vi "ADCP main.vi"() -> ()   [LabVIEW 2016, in "ADCP.lvlib"]
uses:
  ADCP.lvlib
  <vilib>/Utility/config.llb/NI_LVConfig.lvlib
panel:
  out "电压串口号":string
  out "电压通信":bool caption="通信"
  out "错误输出":errorcluster
  out "输出簇":T1
  in  "电压模块设置":bool
  out "显示":T2
  in  "ADCP设置":bool
  out "通信串口号":string
  out "通信":bool
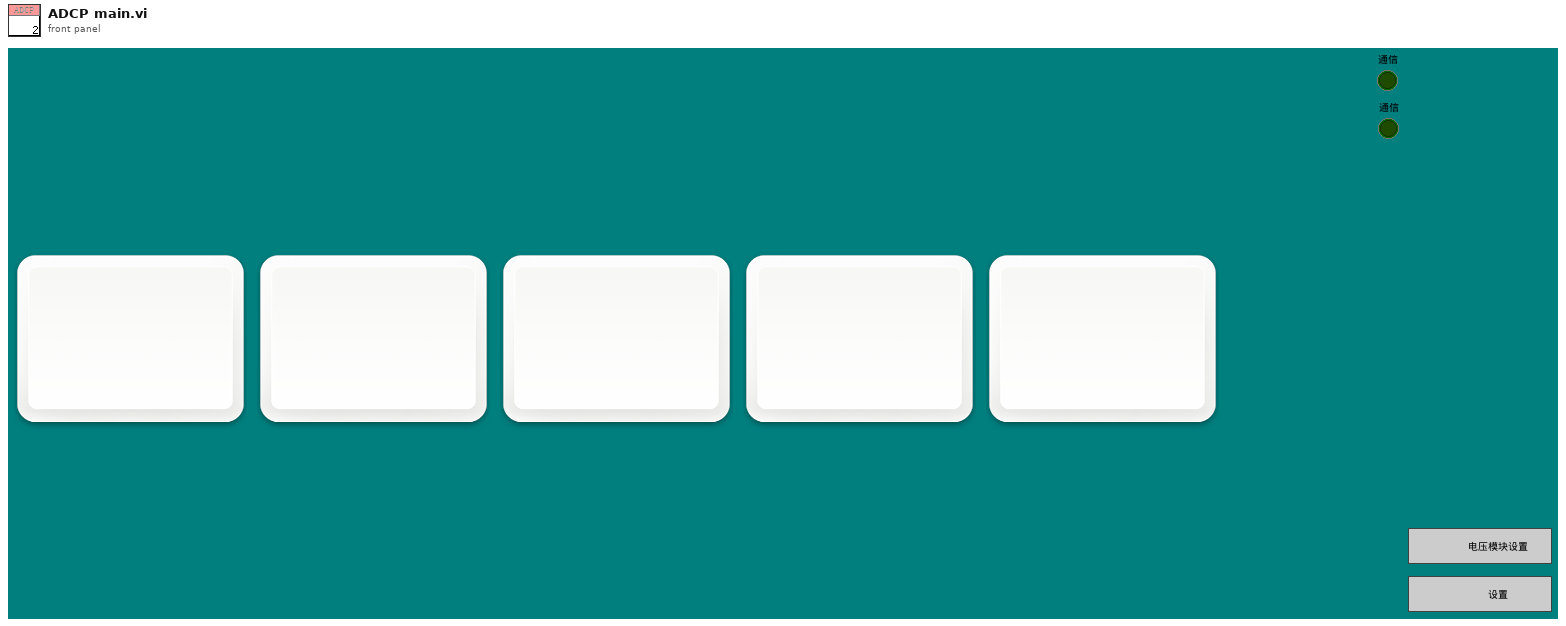
[diagram p1: front panel]
types:
  T1 = cluster{"时间":timestamp, "流速":dbl, "瞬时流量":dbl, "水位":dbl, "正累积流量":dbl, "负累积流量":dbl, "横摇":dbl, "纵摇":dbl, "电压":dbl}
  T2 = typedef "多数值显示.ctl" = cluster{"显示":T3, "显示 2":T3, "显示 3":T3, "显示 4":T3, "显示 5":T3, "显示 6":T3, "显示 12":T3, "显示 11":T3, "显示 10":T3, "显示 9":T3, "显示 8":T3, "显示 7":T3}
  T3 = typedef "数值显示.ctl" = cluster{"中文项目名称":string, "英文项目名称":string, "浓度":string, "单位":string}
  T4 = typedef "NI_LVConfig.lvlib/Config Data RefNum.ctl" = refnum<k1>
  T5 = cluster{"时间":timestamp, "流速":dbl, "瞬时流量":dbl, "方向":string, "水位":dbl, "正累积流量":dbl, "负累积流量":dbl}
  T6 = cluster{"温度":sgl, "水深":sgl, "流速":sgl, "瞬时流量":sgl, "正累积流量":sgl, "负累积流量":sgl, "横滚角":sgl, "俯仰角":sgl}
  T7 = typedef "LVDateTimeRec.ctl" = cluster{"秒数的小数部分":dbl, "秒":i32, "分":i32, "时":i32, "日":i32, "月":i32, "年":i32, "天数（周）":i32, "天数（年）":i32, "DST":i32}
  T8 = cluster{"[0]":sgl, "[1]":sgl, "[2]":sgl, "[3]":sgl, "[4]":sgl, "[5]":sgl}
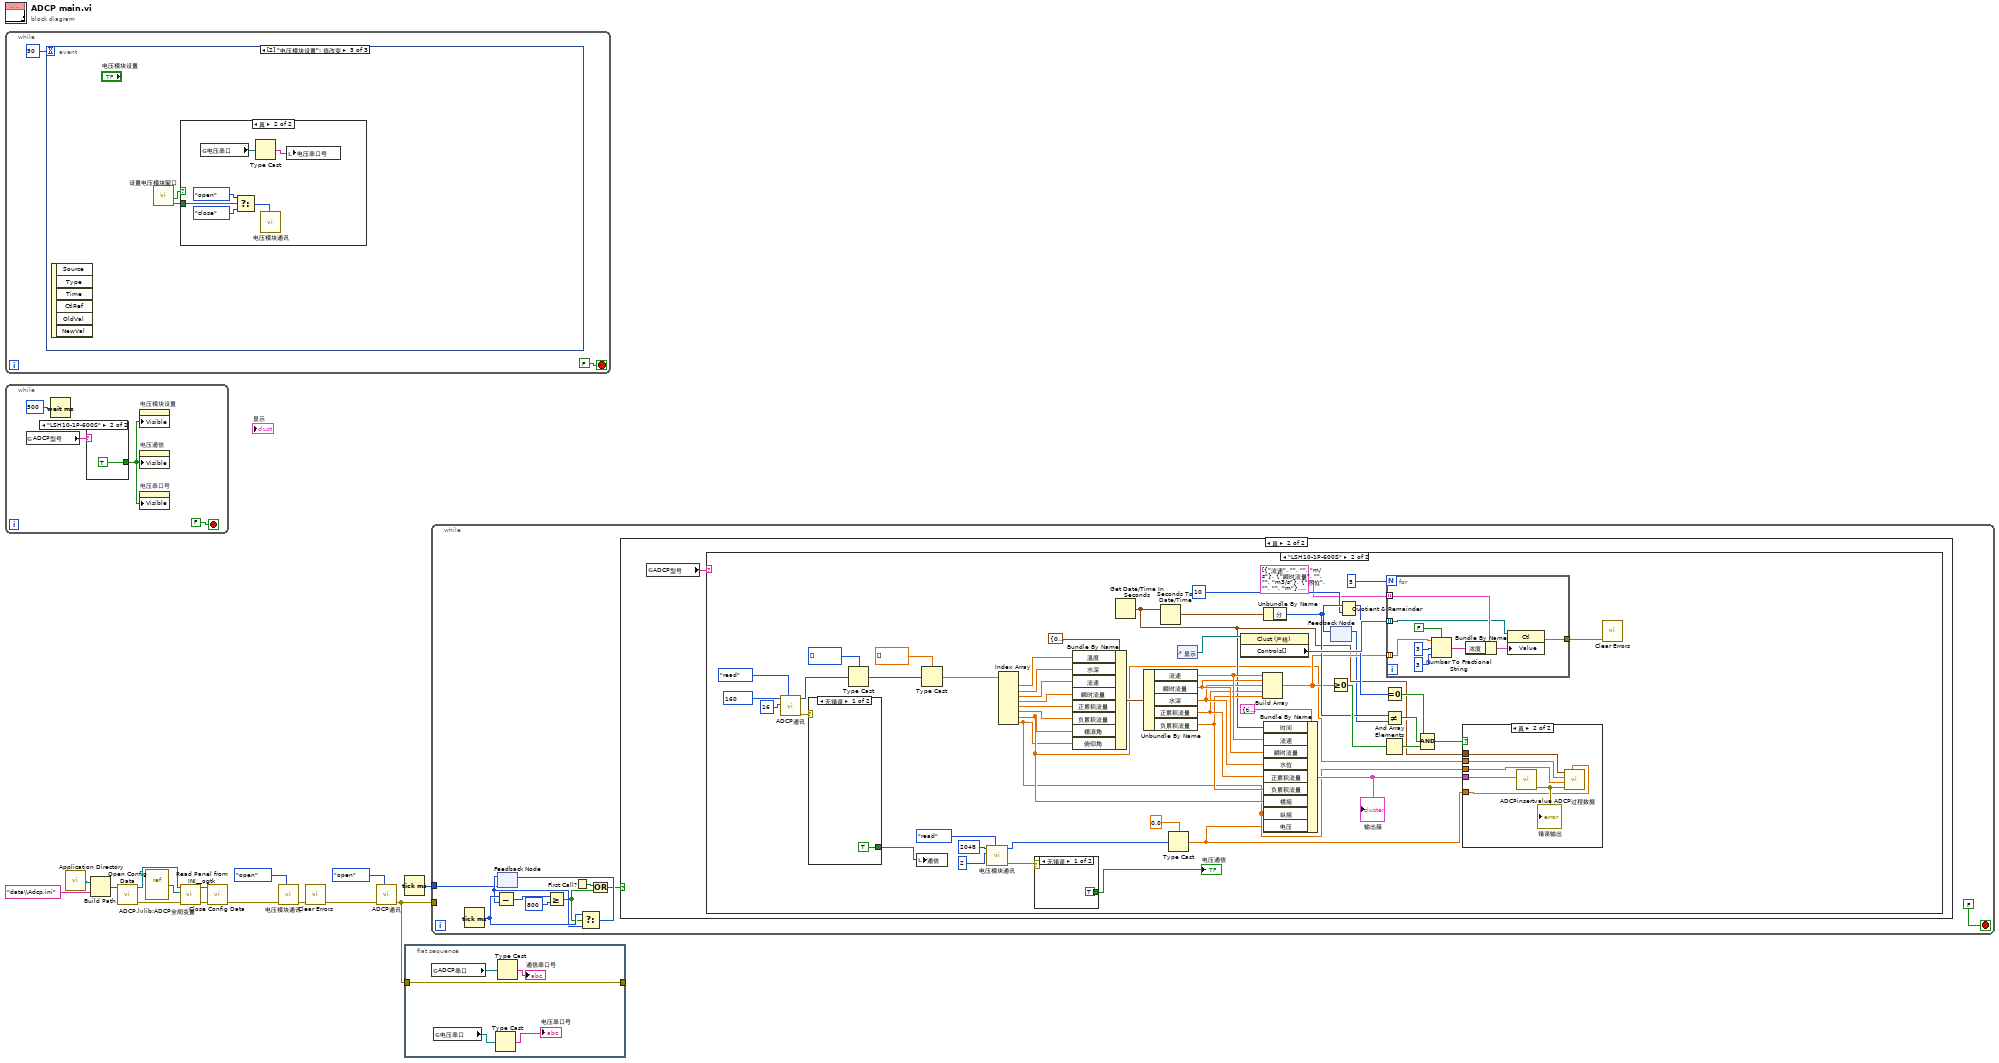
[diagram p0: block diagram]
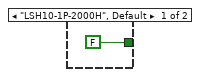
[diagram p2: hidden frame]
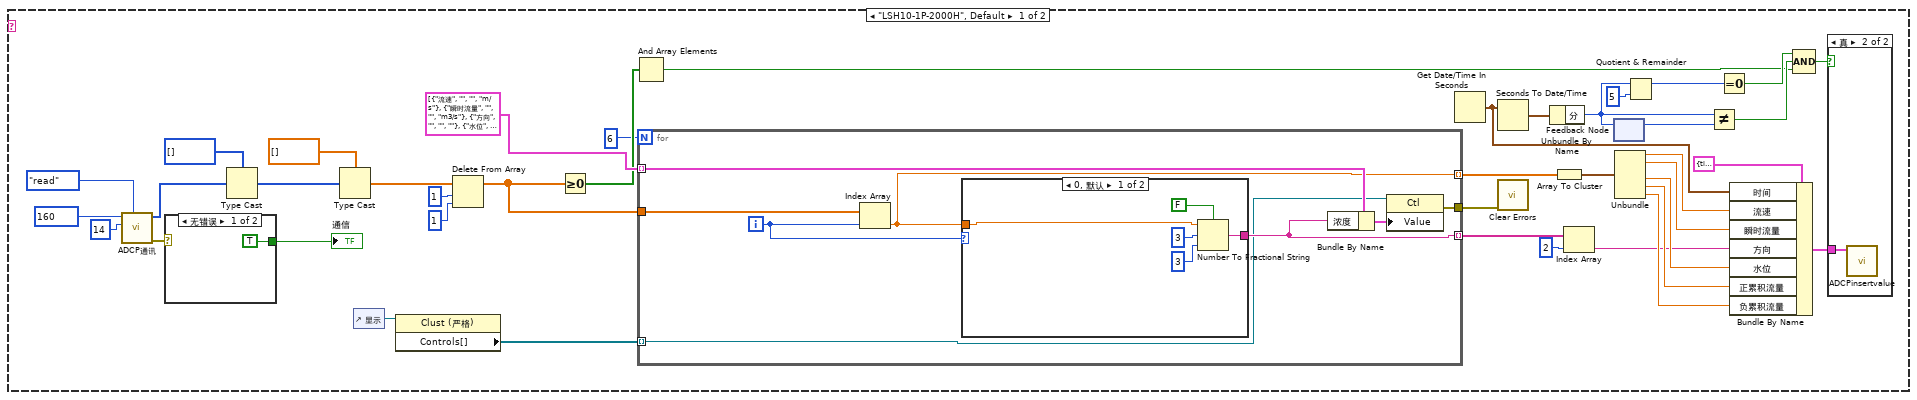
[diagram p4: hidden frame]
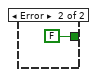
[diagram p5: hidden frame]
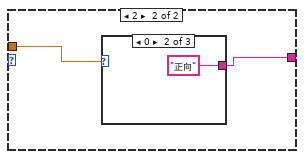
[diagram p7: hidden frame]
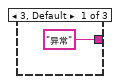
[diagram p8: hidden frame]
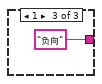
[diagram p9: hidden frame]
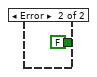
[diagram p10: hidden frame]
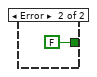
[diagram p11: hidden frame]
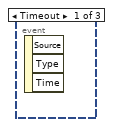
[diagram p13: hidden frame]
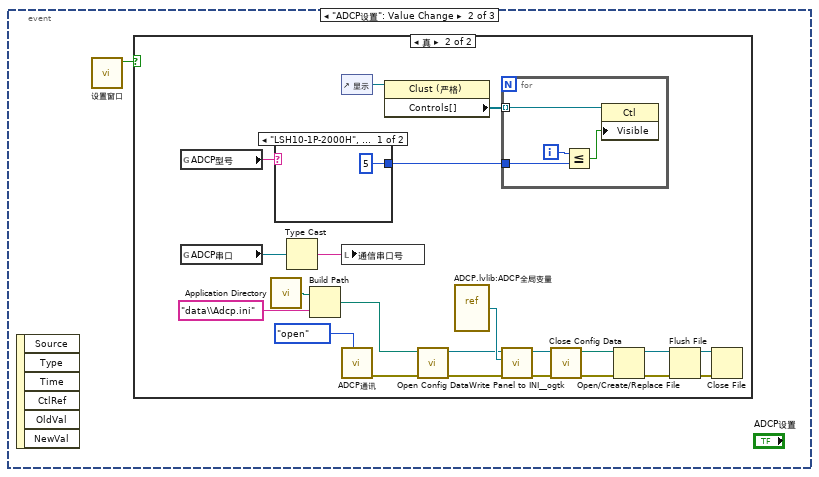
[diagram p14: hidden frame]
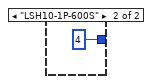
[diagram p16: hidden frame]
diagram:
  n1 = while {
    stop <- FALSE stop-if-true
    n2 = event shown="[2] \"电压模块设置\": 值改变" {
      selector: _ -> [_ _ _]
      dyn-events: _ -> [_ _ _]
      timeout: 50 -> [_ _ _]
      event Timeout {
        n3 = event-data() -> ()  [unwired: 1 in, 3 out]
      }
      event "ADCP设置": Value Change {
        n4 = event-data() -> ()  [unwired: 1 in, 6 out]
        n5 = call "设置窗口.vi"() -> ("确定输出"=w18:bool)  [unwired: 11 in]
        n6 = case shown="真" w18 {
          frame False {
          }
          frame True {
            n7 = global read "ADCP全局变量.vi" "ADCP型号"() -> (w20:string)
            n8 = global read "ADCP全局变量.vi" "ADCP串口"() -> (w24:refnum<visa-resource-name>)
            n9 = call <vilib>:"Application Directory.vi"() -> ("Application Directory"=w27:path)
            n10 = case shown="\"LSH10-1P-2000H\", 默认" w20 {
              tunnel: [5 ("y") 4 ("y")] -> w19
              frame "LSH10-1P-2000H", Default {
              }
              frame "LSH10-1P-600S" {
              }
            }
            n11 = Type Cast(x=w24) -> (*(type *) &x=w25:string)  [unwired: 1 in]
            n12 = Build Path(base path=w27, name or relative path="data\\Adcp.ini" ("名称或相对路径")) -> (appended path=w29:path)
            n13 = control-ref of="显示"() -> (w22:refnum<vi>)
            n14 = local write "通信串口号"(w25) -> ()
            n15 = call "ADCP通讯.vi"("STEP"=enum16{"open", "read", "write", "close"}."open") -> ("error out"=w23:errorcluster)  [unwired: 8 in, 2 out]
            n16 = property class="Clust (严格)"(reference=w22) -> ("Controls[]"=w21:refnum<vi>[])  [unwired: 1 in, 2 out]
            n17 = call <vilib>:"Open Config Data.vi"("error in (no error)"=w23, "configuration file path"=w29) -> ("error out"=w33:errorcluster, "refnum"=w30:T4)  [unwired: 7 in, 1 out]
            n18 = vi-ref "ADCP.lvlib:ADCP全局变量.vi"() -> (w31:refnum<vi>)
            n19 = for {
              tunnel: w21 -> [w44] mode=indexing
              tunnel: w19 -> [w45]
              i -> [w46]
              n20 = Less Or Equal?(x=w46, y=w45) -> (x <= y?=w43:bool)
              n21 = property class="Ctl"(reference=w44, "Visible"=w43) -> ()  [unwired: 1 in, 2 out]
            }
            n22 = call <userlib>:"Write Panel to INI__ogtk.vi"("error in (no error)"=w33, "VI ref"=w31, "refnum"=w30) -> ("error out"=w34:errorcluster, "refnum out"=w32:T4)  [unwired: 7 in]
            n23 = call <vilib>:"Close Config Data.vi"("error in (no error)"=w34, "refnum"=w32) -> ("error out"=w39:errorcluster, "file path"=w40:path)  [unwired: 8 in]
            n24 = Open/Create/Replace File(file path (use dialog)=w40, error in=w39) -> (refnum out=w36:refnum<file>, error out=w35:errorcluster)  [unwired: 4 in, 1 out]
            n25 = Flush File(refnum=w36, error in=w35) -> (refnum out=w37:refnum<file>, error out=w38:errorcluster)
            n26 = Close File(refnum=w37, error in=w38) -> ()  [unwired: 2 out]
          }
        }
      }
      event "电压模块设置": Value Change {
        n27 = event-data() -> ()  [unwired: 1 in, 6 out]
        n28 = call "设置电压模块窗口.vi"() -> ("打开/关闭"=w47:bool, "确定输出"=w48:bool)  [unwired: 10 in]
        n29 = case shown="真" w48 {
          tunnel: w47 -> [_ w54]
          frame False {
          }
          frame True {
            n30 = global read "ADCP全局变量.vi" "电压串口"() -> (w50:refnum<visa-resource-name>)
            n31 = Select(t=enum16{"open", "read", "write", "close"}."open" ("STEP"), s=w54, f=enum16{"open", "read", "write", "close"}."close" ("STEP")) -> (s? t:f=w51:enum16{"open", "read", "write", "close"})
            n32 = Type Cast(x=w50) -> (*(type *) &x=w49:string)  [unwired: 1 in]
            n33 = call "电压模块通讯.vi"("STEP"=w51) -> ()  [unwired: 8 in, 3 out]
            n34 = local write "电压串口号"(w49) -> ()
          }
        }
      }
    }
  }
  n35 = while {
    stop <- FALSE stop-if-true
    n36 = global read "ADCP全局变量.vi" "ADCP型号"() -> (w56:string)
    n37 = Wait (ms)(milliseconds to wait=u32 500 ("等待时间（毫秒）")) -> ()  [unwired: 1 out]
    n38 = case shown="\"LSH10-1P-600S\"" w56 {
      tunnel: [FALSE TRUE] -> w55
      frame "LSH10-1P-2000H", Default {
      }
      frame "LSH10-1P-600S" {
      }
    }
    n39 = property on="电压模块设置" class="Bool"("Visible"=w55) -> ()  [unwired: 2 in, 2 out]
    n40 = property on="电压通信" class="Bool (严格)"("Visible"=w55) -> ()  [unwired: 2 in, 2 out]
    n41 = property on="电压串口号" class="Str"("Visible"=w55) -> ()  [unwired: 2 in, 2 out]
  }
  n42 = call <vilib>:"Application Directory.vi"() -> ("Application Directory"=w10:path)
  n43 = Build Path(base path=w10, name or relative path="data\\Adcp.ini" ("名称或相对路径")) -> (appended path=w12:path)
  n44 = call <vilib>:"Open Config Data.vi"("configuration file path"=w12) -> ("error out"=w8:errorcluster, "refnum"=w13:T4)  [unwired: 8 in, 1 out]
  n45 = vi-ref "ADCP.lvlib:ADCP全局变量.vi"() -> (w7:refnum<vi>)
  n46 = call <userlib>:"Read Panel from INI__ogtk.vi"("error in (no error)"=w8, "VI ref"=w7, "refnum"=w13) -> ("error out"=w9:errorcluster, "refnum out"=w14:T4)  [unwired: 7 in]
  n47 = call <vilib>:"Close Config Data.vi"("error in (no error)"=w9, "refnum"=w14) -> ("error out"=w3:errorcluster)  [unwired: 8 in, 1 out]
  n48 = call "电压模块通讯.vi"("STEP"=enum16{"open", "read", "write", "close"}."open", "Error in"=w3) -> ("error out"=w2:errorcluster)  [unwired: 7 in, 2 out]
  n49 = call <vilib>:"Clear Errors.vi"("error in (no error)"=w2) -> ("error out"=w1:errorcluster)  [unwired: 5 in, 1 out]
  n50 = call "ADCP通讯.vi"("STEP"=enum16{"open", "read", "write", "close"}."open", "Error in"=w1) -> ("error out"=w5:errorcluster)  [unwired: 7 in, 2 out]
  n51 = Tick Count (ms)() -> (millisecond timer value=w6:u32)
  n52 = flat-sequence {
    tunnel: [w63] -> _
    tunnel: w5 -> [w63]
    frame #0 {
      n53 = global read "ADCP全局变量.vi" "ADCP串口"() -> (w64:refnum<visa-resource-name>)
      n54 = global read "ADCP全局变量.vi" "电压串口"() -> (w62:refnum<visa-resource-name>)
      n55 = Type Cast(x=w62) -> (*(type *) &x=→"电压串口号":string)  [unwired: 1 in]
      n56 = Type Cast(x=w64) -> (*(type *) &x=→"通信串口号":string)  [unwired: 1 in]
    }
  }
  n57 = while {
    tunnel: w6 -> [w69]
    tunnel: w5 -> [_]
    stop <- FALSE stop-if-true
    n58 = Tick Count (ms)() -> (millisecond timer value=w72:u32)
    n59 = feedback #1(w69) -> (w71:u32)
    n60 = Subtract(x=w72, y=w71) -> (x-y=w74:u32)
    n61 = Greater Or Equal?(x=w74, y=u32 800) -> (x >= y?=w66:bool)
    n62 = First Call?() -> (First Call?: T/F=w67:bool)
    n63 = Select(t=w72, s=w66, f=w71) -> (s? t:f=w70:u32)
    n64 = feedback-in #1(w70) -> ()
    n65 = Or(x=w67, y=w66) -> (x .or. y?=w68:bool)
    n66 = case shown="真" w68 {
      frame False {
      }
      frame True {
        n67 = global read "ADCP全局变量.vi" "ADCP型号"() -> (w76:string)
        n68 = case shown="\"LSH10-1P-600S\"" w76 {
          frame "LSH10-1P-2000H", Default {
            n69 = call "ADCP通讯.vi"("STEP"=enum16{"open", "read", "write", "close"}."read", "quantity"=u16 14, "starting address"=u16 160) -> ("error out"=w96:errorcluster, "Registers"=w93:u16[])  [unwired: 6 in, 1 out]
            n70 = case shown="无错误" w96 {
              tunnel: [TRUE FALSE] -> w92
              frame No Error {
              }
              frame Error {
              }
            }
            "通信" <- w92
            n71 = Type Cast(type=u32[] [], x=w93) -> (*(type *) &x=w113:u32[])
            n72 = Type Cast(type=sgl[] [], x=w113) -> (*(type *) &x=w111:sgl[])
            n73 = control-ref of="显示"() -> (w117:refnum<vi>)
            n74 = property class="Clust (严格)"(reference=w117) -> ("Controls[]"=w116:refnum<vi>[])  [unwired: 1 in, 2 out]
            n75 = Delete From Array(array=w111, length=1 ("长度"), index=1 ("索引")) -> (array with subset deleted=w79:sgl[])  [unwired: 1 out]
            n76 = Greater Or Equal To 0?(x=w79) -> (x >= 0?=w91:bool[])
            n77 = And Array Elements(Boolean array=w91) -> (logical AND=w83:bool)
            n78 = for {
              N: 6 -> [_]
              tunnel: w116 -> [w125] mode=indexing
              tunnel: T3[] [{"中文项目名称"="流速", "英文项目名称"="", "浓度"="", "单位"="m/s"}, {"中文项目名称"="瞬时流量", "英文项目名称"="", "浓度"="", "单位"="m3/s"}, {"中文项目名称"="方向", "英文项目名称"="", "浓度"="", "单位"=""}, {"中文项目名称"="水位", "英文项目名称"="", "浓度"="", "单位"="m"}, {"中文项目名称"="正累积流量", "英文项目名称"="", "浓度"="", "单位"="m3"}, {"中文项目名称"="负累积流量", "英文项目名称"="", "浓度"="", "单位"="M3"}] -> [w128] mode=indexing
              tunnel: [w126] -> w89 mode=indexing
              tunnel: [w122] -> w90 mode=indexing
              tunnel: w79 -> [w124]
              tunnel: [w121] -> w77
              i -> [w123]
              n79 = Index Array(array=w124, index=w123) -> (element=w122:sgl)
              n80 = case shown="0, 默认" w123 {
                tunnel: [w133 w134] -> w126
                tunnel: w122 -> [w132 w135]
                frame 0, Default {
                  n81 = Number To Fractional String(use system decimal point (T)=FALSE ("使用系统小数点(T)"), number=w132, width (-)=i16 3 ("宽度(-)"), precision (6)=i16 3 ("精度(6)")) -> (F-format string=w133:string)
                }
                frame 2 {
                  n82 = case shown="0" w135 {
                    tunnel: ["异常" "正向" "负向"] -> w134
                    frame 3, Default {
                    }
                    frame 0 {
                    }
                    frame 1 {
                    }
                  }
                }
              }
              n83 = Bundle By Name(cluster=w128, "浓度"=w126) -> (w127:T3)
              n84 = property class="Ctl"(reference=w125, "Value"=w127) -> (error out=w121:errorcluster)  [unwired: 1 in, 1 out]
            }
            n85 = Get Date/Time In Seconds() -> (seconds since 1Jan1904=w99:timestamp)
            n86 = Seconds To Date/Time(time stamp (now)=w99) -> (date time rec=w100:T7)  [unwired: 1 in]
            n87 = call <vilib>:"Clear Errors.vi"("error in (no error)"=w77) -> ()  [unwired: 5 in, 2 out]
            n88 = Unbundle By Name(w100) -> ("分"=w87:i32)
            n89 = Array To Cluster(array=w90) -> (cluster=w107:T8)
            n90 = Index Array(array=w89, index=2 ("索引")) -> (element=w81:string)
            n91 = feedback #2() -> (w101:i32)  [unwired: 1 in]
            n92 = feedback-in #2(w87) -> ()
            n93 = Unbundle(w107) -> ("[0]"=w106:sgl, "[1]"=w105:sgl, "[3]"=w104:sgl, "[4]"=w103:sgl, "[5]"=w102:sgl)  [unwired: 1 out]
            n94 = Quotient & Remainder(x=w87, y=5) -> (x-y*floor(x/y)=w78:i32)  [unwired: 1 out]
            n95 = Not Equal?(x=w87, y=w101) -> (x != y?=w84:bool)
            n96 = Equal To 0?(x=w78) -> (x = 0?=w85:bool)
            n97 = Bundle By Name(cluster=T5 {"时间"=timestamp(3777000960.083023 s since 1904-01-01), "流速"=0.0, "瞬时流量"=0.0, "方向"="", "水位"=0.0, "正累积流量"=0.0, "负累积流量"=0.0} ("输出簇"), "时间"=w99, "流速"=w106, "瞬时流量"=w105, "方向"=w81, "水位"=w104, "正累积流量"=w103, "负累积流量"=w102) -> (w98:T5)
            n98 = Compound Arithmetic op=AND ("复合运算")(w85, w84, w83) -> (w82:bool)
            n99 = case shown="真" w82 {
              tunnel: w98 -> [_ w120]
              frame False {
              }
              frame True {
                n100 = call "ADCPinsertvalue.vi"("2000H数据"=w120) -> ()  [unwired: 10 in, 1 out]
              }
            }
          }
          frame "LSH10-1P-600S" {
            n101 = call "ADCP通讯.vi"("STEP"=enum16{"open", "read", "write", "close"}."read", "quantity"=u16 16, "starting address"=u16 160) -> ("error out"=w182:errorcluster, "Registers"=w179:u16[])  [unwired: 6 in, 1 out]
            n102 = case shown="无错误" w182 {
              tunnel: [TRUE FALSE] -> w152
              frame No Error {
              }
              frame Error {
              }
            }
            n103 = Type Cast(type=u32[] [], x=w179) -> (*(type *) &x=w186:u32[])
            n104 = local write "通信"(w152) -> ()
            n105 = Type Cast(type=sgl[] [], x=w186) -> (*(type *) &x=w167:sgl[])
            n106 = call "电压模块通讯.vi"("STEP"=enum16{"open", "read", "write", "close"}."read", "quantity"=u16 2, "starting address"=u16 2048) -> ("error out"=w140:errorcluster, "Registers"=w144:u16[])  [unwired: 6 in, 1 out]
            n107 = Index Array(array=w167) -> (element #1=w166:sgl, element #2=w165:sgl, element #3=w164:sgl, element #4=w163:sgl, element #5=w162:sgl, element #6=w161:sgl, element #7=w149:sgl, element #8=w148:sgl)  [unwired: 8 in]
            n108 = case shown="无错误" w140 {
              tunnel: [TRUE FALSE] -> w139
              frame No Error {
              }
              frame Error {
              }
            }
            "电压通信" <- w139
            n109 = Bundle By Name(cluster=T6 {"温度"=0.0, "水深"=0.0, "流速"=0.0, "瞬时流量"=0.0, "正累积流量"=0.0, "负累积流量"=0.0, "横滚角"=0.0, "俯仰角"=0.0} ("运行参数"), "温度"=w166, "水深"=w165, "流速"=w164, "瞬时流量"=w163, "正累积流量"=w162, "负累积流量"=w161, "横滚角"=w149, "俯仰角"=w148) -> (w160:T6)
            n110 = Get Date/Time In Seconds() -> (seconds since 1Jan1904=w151:timestamp)
            n111 = Unbundle By Name(w160) -> ("流速"=w157:sgl, "瞬时流量"=w156:sgl, "水深"=w155:sgl, "正累积流量"=w154:sgl, "负累积流量"=w153:sgl)
            n112 = Seconds To Date/Time(time stamp (now)=w151) -> (date time rec=w185:T7)  [unwired: 1 in]
            n113 = Type Cast(type=sgl 0.0, x=w144) -> (*(type *) &x=w142:sgl)
            n114 = control-ref of="显示"() -> (w190:refnum<vi>)
            n115 = property class="Clust (严格)"(reference=w190) -> ("Controls[]"=w189:refnum<vi>[])  [unwired: 1 in, 2 out]
            n116 = Build Array(w157, w156, w155, w154, w153) -> (w159:sgl[])
            n117 = Unbundle By Name(w185) -> ("分"=w177:i32)
            n118 = Bundle By Name(cluster=T1 {"时间"=timestamp(3777000960.083023 s since 1904-01-01), "流速"=0.0, "瞬时流量"=0.0, "水位"=0.0, "正累积流量"=0.0, "负累积流量"=0.0, "横摇"=0.0, "纵摇"=0.0, "电压"=0.0} ("输出簇"), "时间"=w151, "流速"=w157, "瞬时流量"=w156, "水位"=w155, "正累积流量"=w154, "负累积流量"=w153, "横摇"=w149, "纵摇"=w148, "电压"=w142) -> (w184:T1)
            "输出簇" <- w184
            n119 = Greater Or Equal To 0?(x=w159) -> (x >= 0?=w178:bool[])
            n120 = feedback #3() -> (w141:i32)  [unwired: 1 in]
            n121 = feedback-in #3(w177) -> ()
            n122 = Quotient & Remainder(x=w177, y=10) -> (x-y*floor(x/y)=w170:i32)  [unwired: 1 out]
            n123 = Equal To 0?(x=w170) -> (x = 0?=w175:bool)
            n124 = Not Equal?(x=w177, y=w141) -> (x != y?=w174:bool)
            n125 = And Array Elements(Boolean array=w178) -> (logical AND=w173:bool)
            n126 = for {
              N: 5 -> [_]
              tunnel: w189 -> [w207] mode=indexing
              tunnel: T3[] [{"中文项目名称"="流速", "英文项目名称"="", "浓度"="", "单位"="m/s"}, {"中文项目名称"="瞬时流量", "英文项目名称"="", "浓度"="", "单位"="m3/s"}, {"中文项目名称"="水位", "英文项目名称"="", "浓度"="", "单位"="m"}, {"中文项目名称"="正累积流量", "英文项目名称"="", "浓度"="", "单位"="m3"}, {"中文项目名称"="负累积流量", "英文项目名称"="", "浓度"="", "单位"="M3"}] -> [w209] mode=indexing
              tunnel: w159 -> [w202] mode=indexing
              tunnel: [w206] -> w169
              n127 = Number To Fractional String(use system decimal point (T)=FALSE ("使用系统小数点(T)"), number=w202, width (-)=i16 3 ("宽度(-)"), precision (6)=i16 3 ("精度(6)")) -> (F-format string=w201:string)
              n128 = Bundle By Name(cluster=w209, "浓度"=w201) -> (w208:T3)
              n129 = property class="Ctl"(reference=w207, "Value"=w208) -> (error out=w206:errorcluster)  [unwired: 1 in, 1 out]
            }
            n130 = Compound Arithmetic op=AND ("复合运算")(w175, w174, w173) -> (w172:bool)
            n131 = case shown="真" w172 {
              tunnel: w184 -> [_ w195]
              tunnel: w151 -> [_ w199]
              tunnel: w149 -> [_ w198]
              tunnel: w148 -> [_ w197]
              tunnel: w142 -> [_ w196]
              frame False {
              }
              frame True {
                n132 = call "ADCPinsertvalue.vi"("600S数据"=w195) -> ("错误输出"=w200:errorcluster)  [unwired: 10 in]
                "错误输出" <- w200
                n133 = call "ADCP过程数据.vi"("电压"=w196, "Error in"=w200, "纵摇"=w197, "横摇"=w198, "时间"=w199) -> ()  [unwired: 6 in, 1 out]
              }
            }
            n134 = call <vilib>:"Clear Errors.vi"("error in (no error)"=w169) -> ()  [unwired: 5 in, 2 out]
          }
        }
      }
    }
  }
